vi "CheckFileExist.vi"(0 "Path":string, 1 "error in (no error)":errorcluster) -> (2 "Exist":bool, 3 "Overwrite":bool, 4 "error out":errorcluster)   [LabVIEW 2009]
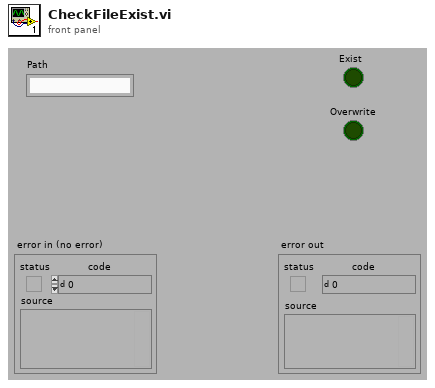
[diagram p1: front panel]
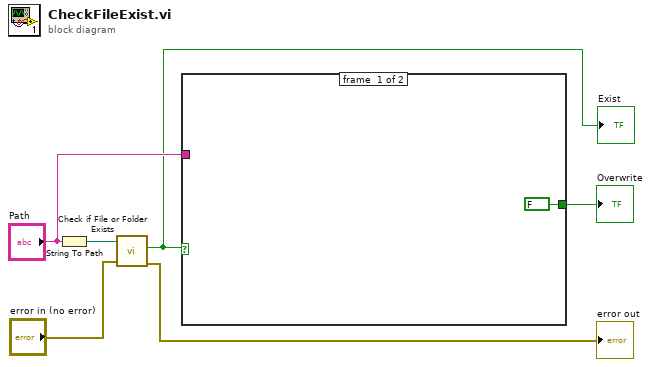
[diagram p0: block diagram]
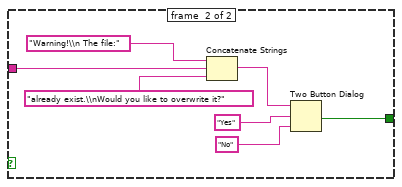
[diagram p2: hidden frame]
diagram:
  n1 = String To Path(string="Path") -> (path=w6:path)
  n2 = call <vilib>:"Check if File or Folder Exists.vi"("error in (no error)"="error in (no error)", "path"=w6) -> ("error out"=→"error out":errorcluster, "file or folder exists?"=w2:bool)  [unwired: 7 in, 1 out]
  "Exist" <- w2
  n3 = case shown="False" w2 {
    tunnel: "Path" -> [_ w12]
    tunnel: [FALSE ("T button?") w8] -> w1
    frame #0 {
    }
    frame #1 {
      n4 = Concatenate Strings("Warning!\\n The file:", w12, "already exist.\\nWould you like to overwrite it?") -> (w11:string)
      n5 = Two Button Dialog(message=w11, 1:"No" ("Right Button Text (\"Cancel\")"), 2:"Yes" ("Right Button Text (\"Cancel\")")) -> (T button?=w8:bool)
    }
  }
  "Overwrite" <- w1
